vi "CRYAPI SPLITE LIB.vi"(4 "tSpliter_In":T3, 6 "tFrame":T2, 8 "tSpliter":T3, 9 "sData":string, 10 "nData":i32, 11 "sAction":string) -> (0 "nData_Out":i32, 2 "tFrame_Out":T2, 3 "tSpliter_Out":T3)   [LabVIEW 2013]
uses:
  <vilib>/Utility/miscctls.llb/LVRectTypeDef.ctl
  CRYMain Sub Window Global.vi
panel:
  out "sData_Out":string
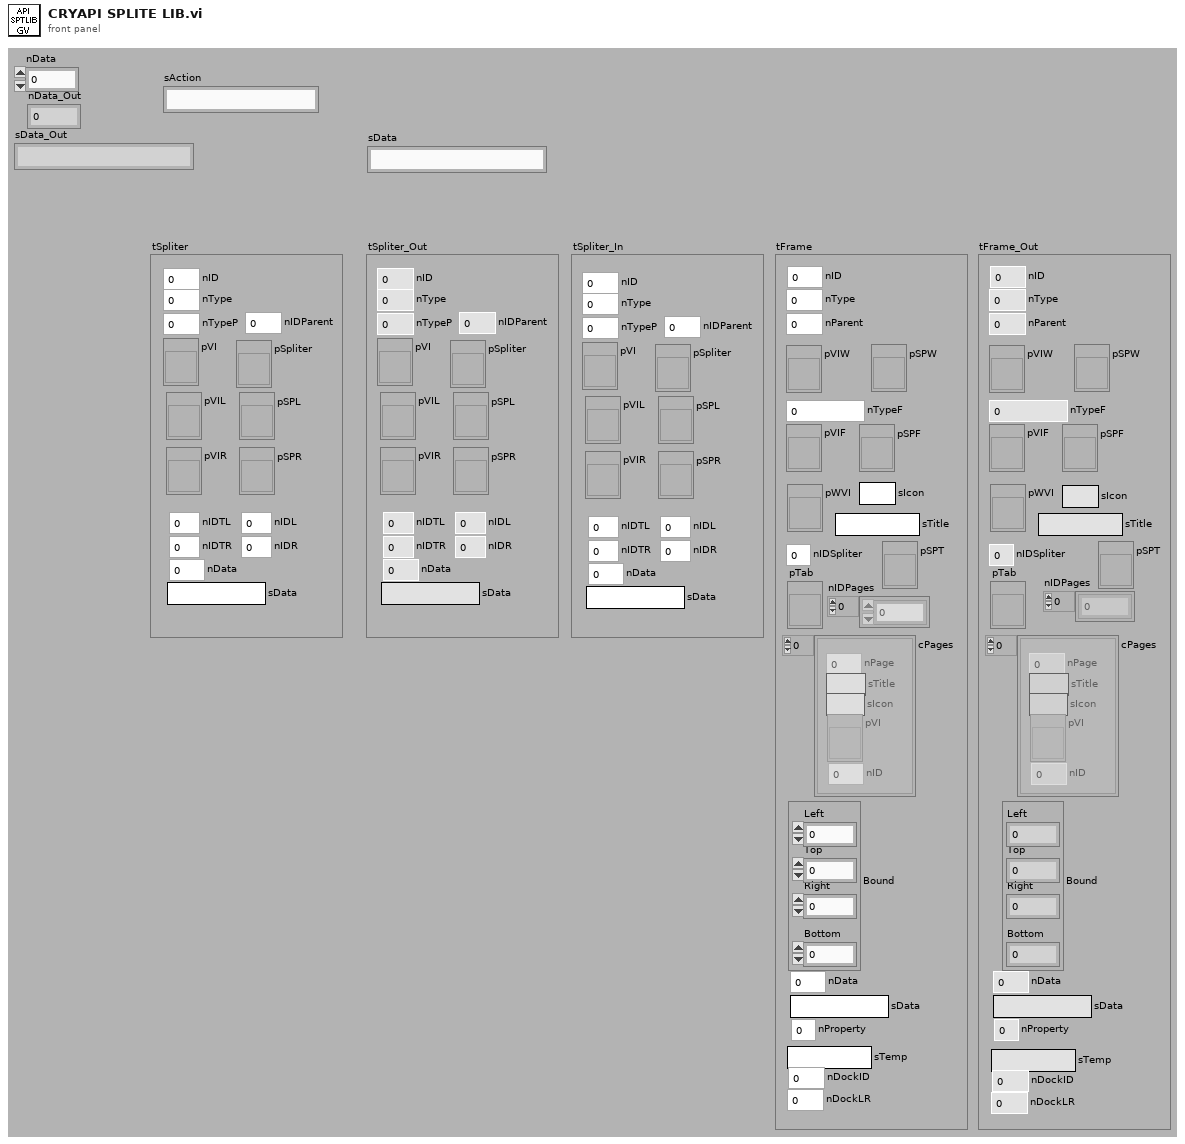
[diagram p1: front panel]
types:
  T1 = typedef "LVRectTypeDef.ctl" = cluster{"Left":i16, "Top":i16, "Right":i16, "Bottom":i16}
  T2 = cluster{"nType":i32, "nParent":i32, "pVIW":refnum<vi>, "pSPW":refnum<vi>, "nTypeF":i32, "pVIF":refnum<vi>, "pSPF":refnum<vi>, "nIDSpliter":i32, "nProperty":i32, "Bound":T1, "nID":i32, "nData":i32, "sData":string, "pWVI":refnum<vi>, "sTitle":string, "cPages":cluster{"nPage":i32, "sTitle":string, "sIcon":string, "pVI":refnum<vi>, "nID":i32}[], "pTab":refnum<vi>, "nIDPages":i32[], "pSPT":refnum<vi>, "sTemp":string, "nDockID":i32, "nDockLR":i32, "sIcon":string}
  T3 = cluster{"nType":i32, "nTypeP":i32, "pVI":refnum<vi>, "pSpliter":refnum<vi>, "pSPL":refnum<vi>, "pVIL":refnum<vi>, "pSPR":refnum<vi>, "pVIR":refnum<vi>, "nIDTL":i32, "nIDL":i32, "nIDTR":i32, "nIDR":i32, "nID":i32, "nIDParent":i32, "nData":i32, "sData":string}
  T4 = enum16{"Sticks Top/Left", "Sticks Bottom/Right", "Proportional"}
  T5 = enum32{"Invalid", "Standard", "Closed", "Hidden", "Minimized", "Maximized"}
  T6 = cluster{"pSP":refnum<vi>, "pVI":refnum<vi>, "nIDT":i32, "nID":i32, "nLR":i32}
  T7 = typedef "LVBoundsTypeDef.ctl" = cluster{"Width":u32, "Height":u32}
  T8 = cluster{"nID":i32[], "Spliter":cluster{"nType":i32, "nTypeP":i32, "pVI":refnum<vi>, "pSpliter":refnum<vi>, "pSPL":refnum<vi>, "pVIL":refnum<vi>, "pSPR":refnum<vi>, "pVIR":refnum<vi>, "nIDTL":i32, "nIDL":i32, "nIDTR":i32, "nIDR":i32, "nID":i32, "nIDParent":i32, "nData":i32, "sData":string}[]}
  T9 = cluster{"nType":i32, "nTypeP":i32, "pVI":refnum<vi>, "pSpliter":refnum<vi>, "pSPL":refnum<vi>, "pVIL":refnum<vi>, "pSPR":refnum<vi>, "pVIR":refnum<vi>, "nIDTL":i32, "nIDL":i32, "nIDTR":i32, "nIDR":i32, "nID":i32, "nIDParent":i32, "nData":i32, "sData":string}[]
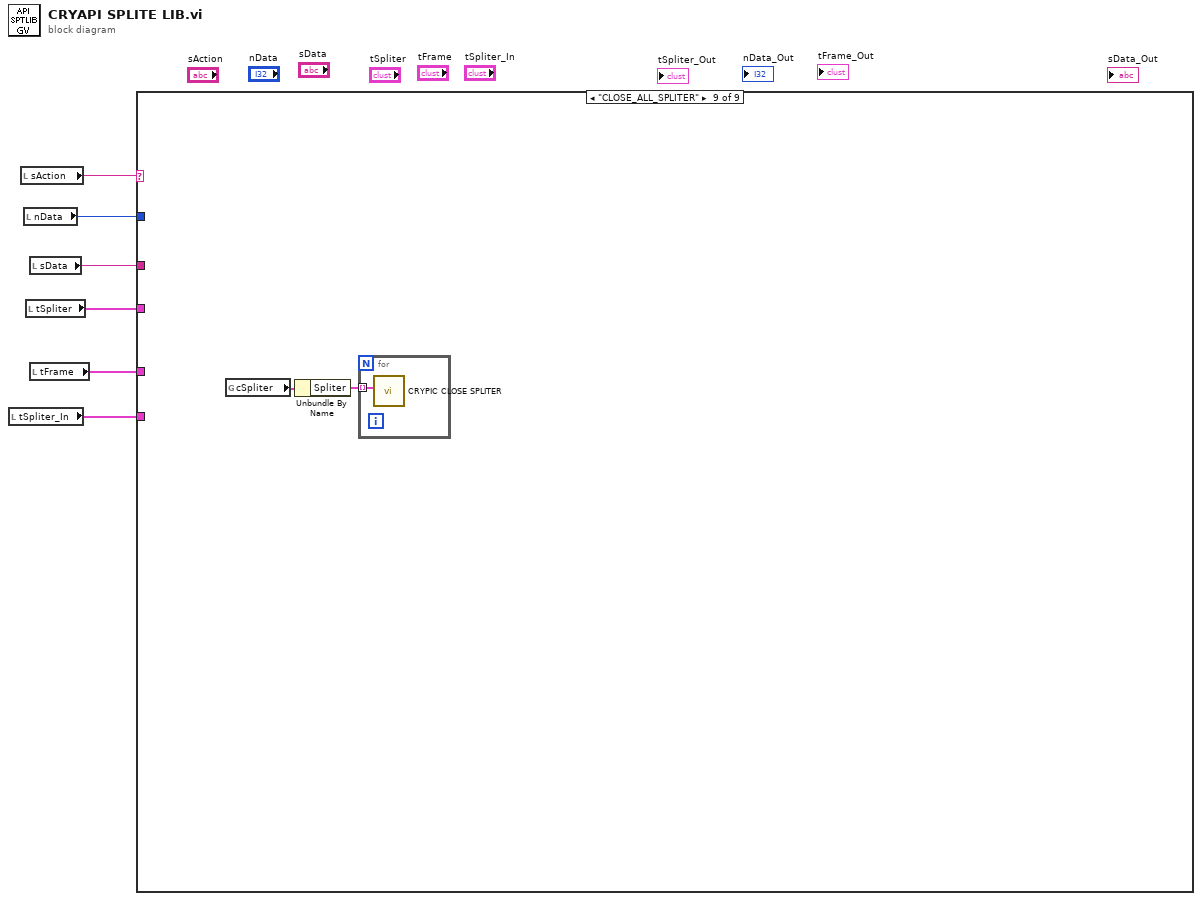
[diagram p0: block diagram]
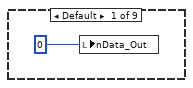
[diagram p2: hidden frame]
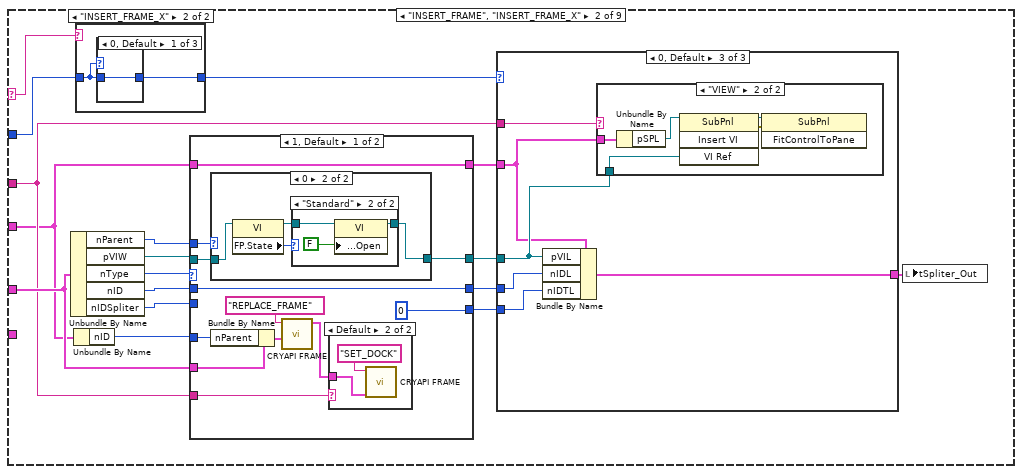
[diagram p3: hidden frame]
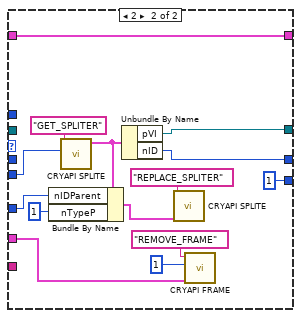
[diagram p7: hidden frame]
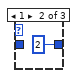
[diagram p9: hidden frame]
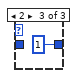
[diagram p10: hidden frame]
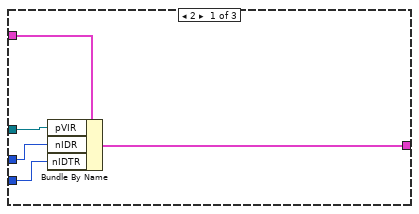
[diagram p11: hidden frame]
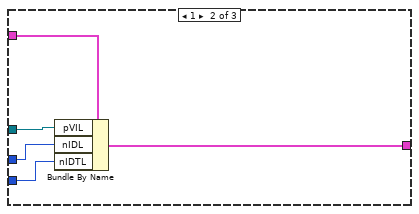
[diagram p12: hidden frame]
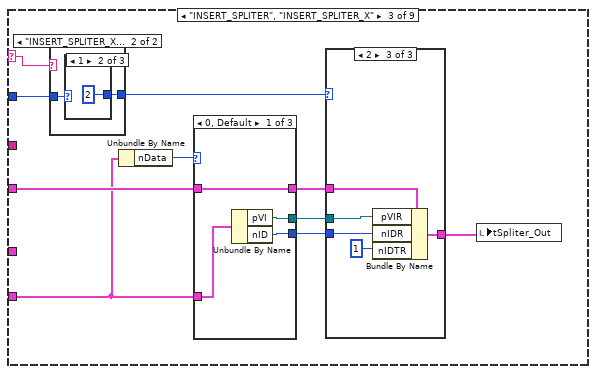
[diagram p14: hidden frame]
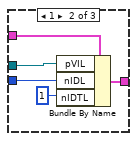
[diagram p16: hidden frame]
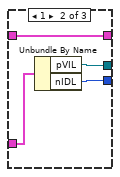
[diagram p17: hidden frame]
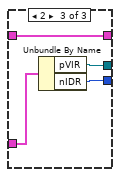
[diagram p18: hidden frame]
diagram:
  n1 = local read "tSpliter_In"() -> (w2:T3)
  n2 = local read "sAction"() -> (w6:string)
  n3 = local read "nData"() -> (w5:i32)
  n4 = local read "tSpliter"() -> (w1:T3)
  n5 = local read "sData"() -> (w3:string)
  n6 = local read "tFrame"() -> (w4:T2)
  n7 = case shown="\"CLOSE_ALL_SPLITER\"" w6 {
    selector: w6 -> [_ w16 w96 _ _ _ _ _ _]
    tunnel: w1 -> [_ w9 w97 w128 _ w391 _ _ _]
    tunnel: w5 -> [_ w15 w98 w130 w289 w392 w473 _ _]
    tunnel: w4 -> [_ w14 _ _ w291 w390 _ _ _]
    tunnel: w3 -> [_ w11 _ _ w290 _ _ _ _]
    tunnel: w2 -> [_ _ w90 w129 _ _ _ _ _]
    frame Default {
      n8 = local write "nData_Out"(0 ("nData_Out")) -> ()
    }
    frame "INSERT_FRAME", "INSERT_FRAME_X" {
      n9 = Unbundle By Name(w14) -> ("nParent"=w8:i32, "pVIW"=w12:refnum<vi>, "nType"=w22:i32, "nID"=w21:i32, "nIDSpliter"=w17:i32)
      n10 = Unbundle By Name(w9) -> ("nID"=w10:i32)
      n11 = case shown="\"INSERT_FRAME_X\"" w16 {
        tunnel: w15 -> [w62 w63]
        tunnel: [w62 w64] -> w23
        frame Default {
        }
        frame "INSERT_FRAME_X" {
          n12 = case shown="0, Default" w63 {
            tunnel: [w65 2 ("nData") 1 ("nData")] -> w64
            tunnel: w63 -> [w65 _ _]
            frame 0, Default {
            }
            frame 1 {
            }
            frame 2 {
            }
          }
        }
      }
      n13 = case shown="1, Default" w22 {
        tunnel: w21 -> [w32 _]
        tunnel: [w25 w58] -> w20
        tunnel: [w32 w57] -> w19
        tunnel: [0 ("nIDTR") 1 ("nIDTR")] -> w18
        tunnel: w17 -> [_ w59]
        tunnel: w14 -> [w33 w48]
        tunnel: w9 -> [w35 w54]
        tunnel: [w35 w54] -> w13
        tunnel: w10 -> [w31 w52]
        tunnel: w12 -> [w34 _]
        tunnel: w11 -> [w27 _]
        tunnel: w8 -> [w26 _]
        frame 1, Default {
          n14 = case shown="0" w26 {
            tunnel: w34 -> [w37 w39]
            tunnel: [w37 w38] -> w25
            frame Default {
            }
            frame 0 {
              n15 = property class="VI"(reference=w39) -> (reference out=w41:refnum<vi>, "FP.State"=w40:T5)  [unwired: 1 in, 1 out]
              n16 = case shown="\"Standard\"" w40 {
                tunnel: w41 -> [w42 w45]
                tunnel: [w42 w43] -> w38
                frame "Invalid", Default {
                }
                frame "Standard" {
                  n17 = property class="VI"(reference=w45, "Front Panel.Open"=FALSE ("Front Panel Window:Open")) -> (reference out=w43:refnum<vi>)  [unwired: 1 in, 1 out]
                }
              }
            }
          }
          n18 = Bundle By Name(cluster=w33, "nParent"=w31) -> (w29:T2)
          n19 = call "CRYAPI FRAME.vi"("tFrame"=w29, "sAction"="REPLACE_FRAME") -> ("tFrame_Out"=w28:T2)  [unwired: 4 in, 5 out]
          n20 = case shown="Default" w27 {
            tunnel: w28 -> [_ w46]
            frame "VIEW" {
            }
            frame Default {
              n21 = call "CRYAPI FRAME.vi"("tFrame"=w46, "sAction"="SET_DOCK") -> ()  [unwired: 4 in, 6 out]
            }
          }
        }
        frame 2 {
          n22 = call "CRYAPI SPLITE.vi"("nData"=w59, "sAction"="GET_SPLITER") -> ("tSpliter_Out"=w53:T3)  [unwired: 4 in, 5 out]
          n23 = Bundle By Name(cluster=w53, "nIDParent"=w52, "nTypeP"=1) -> (w49:T3)
          n24 = Unbundle By Name(w53) -> ("pVI"=w58:refnum<vi>, "nID"=w57:i32)
          n25 = call "CRYAPI SPLITE.vi"("tSpliter"=w49, "sAction"="REPLACE_SPLITER") -> ()  [unwired: 4 in, 6 out]
          n26 = call "CRYAPI FRAME.vi"("tFrame"=w48, "nData"=1, "sAction"="REMOVE_FRAME") -> ()  [unwired: 3 in, 6 out]
        }
      }
      n27 = case shown="0, Default" w23 {
        tunnel: [w72 w77 w81] -> w24
        tunnel: w20 -> [w71 w76 w79]
        tunnel: w19 -> [w70 w75 w83]
        tunnel: w18 -> [w68 w74 w82]
        tunnel: w13 -> [w69 w73 w78]
        tunnel: w11 -> [_ _ w80]
        frame 2 {
          n28 = Bundle By Name(cluster=w69, "pVIR"=w71, "nIDR"=w70, "nIDTR"=w68) -> (w72:T3)
        }
        frame 1 {
          n29 = Bundle By Name(cluster=w73, "pVIL"=w76, "nIDL"=w75, "nIDTL"=w74) -> (w77:T3)
        }
        frame 0, Default {
          n30 = Bundle By Name(cluster=w78, "pVIL"=w79, "nIDL"=w83, "nIDTL"=w82) -> (w81:T3)
          n31 = case shown="\"VIEW\"" w80 {
            tunnel: w79 -> [_ w84]
            tunnel: w78 -> [_ w88]
            frame Default {
            }
            frame "VIEW" {
              n32 = Unbundle By Name(w88) -> ("pSPL"=w87:refnum<vi>)
              n33 = invoke class="SubPnl" method="Insert VI"(reference=w87, "VI Ref"=w84) -> (reference out=w86:refnum<vi>, error out=w85:errorcluster)  [unwired: 2 in, 2 out]
              n34 = invoke class="SubPnl" method="FitControlToPane"(reference=w86, error in=w85) -> ()  [unwired: 1 in, 3 out]
            }
          }
        }
      }
      n35 = local write "tSpliter_Out"(w24) -> ()
    }
    frame "INSERT_SPLITER", "INSERT_SPLITER_X" {
      n36 = case shown="\"INSERT_SPLITER_X\"" w96 {
        tunnel: w98 -> [w122 w124]
        tunnel: [w122 w123] -> w95
        frame "INSERT_SPLITER", Default {
        }
        frame "INSERT_SPLITER_X" {
          n37 = case shown="1" w124 {
            selector: w124 -> [w125 _ _]
            tunnel: [w125 2 ("nData") 1 ("nData")] -> w123
            frame 0, Default {
            }
            frame 1 {
            }
            frame 2 {
            }
          }
        }
      }
      n38 = Unbundle By Name(w90) -> ("nData"=w89:i32)
      n39 = case shown="0, Default" w89 {
        tunnel: w97 -> [w112 w116 w120]
        tunnel: w90 -> [w113 w117 w121]
        tunnel: [w112 w116 w120] -> w94
        tunnel: [w111 w115 w119] -> w93
        tunnel: [w110 w114 w118] -> w92
        frame 0, Default {
          n40 = Unbundle By Name(w113) -> ("pVI"=w111:refnum<vi>, "nID"=w110:i32)
        }
        frame 1 {
          n41 = Unbundle By Name(w117) -> ("pVIL"=w115:refnum<vi>, "nIDL"=w114:i32)
        }
        frame 2 {
          n42 = Unbundle By Name(w121) -> ("pVIR"=w119:refnum<vi>, "nIDR"=w118:i32)
        }
      }
      n43 = case shown="2" w95 {
        tunnel: w94 -> [w99 w104 w109]
        tunnel: w93 -> [_ w102 w107]
        tunnel: w92 -> [_ w101 w106]
        tunnel: [w99 w100 w105] -> w91
        frame 0, Default {
        }
        frame 1 {
          n44 = Bundle By Name(cluster=w104, "pVIL"=w102, "nIDL"=w101, "nIDTL"=1) -> (w100:T3)
        }
        frame 2 {
          n45 = Bundle By Name(cluster=w109, "pVIR"=w107, "nIDR"=w106, "nIDTR"=1 ("nIDTL")) -> (w105:T3)
        }
      }
      n46 = local write "tSpliter_Out"(w91) -> ()
    }
    frame "MSIZE_SPLITER" {
      n47 = local write "tSpliter_Out"(w128) -> ()
      n48 = stacked-sequence {
        tunnel: w130 -> [w153 w250]
        tunnel: w129 -> [_ w261]
        tunnel: w128 -> [w152 w253]
        tunnel: w128 -> [w134 _]
        frame #0 {
          n49 = global read "CRYMain Sub Window Global.vi" "VritualVI"() -> (w138:refnum<vi>)
          n50 = Unbundle By Name(w134) -> ("nIDTL"=w133:i32, "nIDTR"=w132:i32)
          n51 = Unbundle By Name(w152) -> ("pVI"=w140:refnum<vi>)
          n52 = call "CRYAPI SPLITE.vi"("tSpliter"=w152, "nData"=w153, "sAction"="GET_LR_INDEX") -> ("tLR_Out"=w136:T6)  [unwired: 3 in, 5 out]
          n53 = Unbundle By Name(w136) -> ("pSP"=w135:refnum<vi>)
          n54 = Add(x=w133, y=w132) -> (x+y=w131:i32)
          n55 = property class="VI"(reference=w140) -> ("Front Panel.PanelBounds"=w139:T1)  [unwired: 1 in, 2 out]
          n56 = property class="VI"(reference=w138) -> ("Front Panel.PanelBounds"=w150:T1)  [unwired: 1 in, 2 out]
          n57 = property class="SubPnl"(reference=w135) -> ("Bounds"=w137:T7)  [unwired: 1 in, 2 out]
          n58 = Unbundle By Name(w152) -> ("nType"=w149:i32, "pSpliter"=w142:refnum<vi>)
          n59 = Unbundle By Name(w136) -> ("nIDT"=w147:i32)
          n60 = case shown="0, 1, Default" w149 {
            tunnel: w150 -> [w200 w225]
            tunnel: [w190 w215] -> w145
            tunnel: [w186 w211] -> w144
            tunnel: [w199 w224] -> w143
            tunnel: w153 -> [w198 w223]
            tunnel: [w198 w223] -> w148
            tunnel: w147 -> [w197 w222]
            tunnel: [w197 w222] -> w146
            tunnel: w142 -> [w196 w216]
            tunnel: [w196 w216] -> w141
            tunnel: w139 -> [w191 w217]
            tunnel: w137 -> [w189 w213]
            tunnel: w131 -> [w187 w212]
            frame 2 {
              n61 = Unbundle By Name(w200) -> ("Right"=w201:i16, "Left"=w202:i16, "Bottom"=w203:i16, "Top"=w204:i16)
              n62 = Unbundle By Name(w191) -> ("Right"=w195:i16, "Left"=w194:i16, "Bottom"=w193:i16, "Top"=w192:i16)
              n63 = Subtract(x=w201, y=w202) -> ()  [unwired: 1 out]
              n64 = Subtract(x=w203, y=w204) -> (x-y=w186:i16)
              n65 = case shown="Default" w187 {
                tunnel: w189 -> [_ w210]
                tunnel: [w206 w209] -> w188
                tunnel: w186 -> [w208 _]
                frame 0 {
                  n66 = Divide(x=w208, y=i16 2) -> (x/y=w205:dbl)
                  n67 = To Long Integer(number=w205) -> (32bit integer=w206:i32)
                }
                frame Default {
                  n68 = Unbundle By Name(w210) -> ("Height"=w209:u32)  [unwired: 1 out]
                }
              }
              n69 = Subtract(x=w195, y=w194) -> ()  [unwired: 1 out]
              n70 = Subtract(x=w193, y=w192) -> (x-y=w190:i16)
              n71 = Add(x=w186, y=w188) -> (x+y=w199:u32)
            }
            frame 0, 1, Default {
              n72 = Unbundle By Name(w225) -> ("Right"=w226:i16, "Left"=w227:i16, "Bottom"=w228:i16, "Top"=w229:i16)
              n73 = Unbundle By Name(w217) -> ("Right"=w221:i16, "Left"=w220:i16, "Bottom"=w219:i16, "Top"=w218:i16)
              n74 = Subtract(x=w226, y=w227) -> (x-y=w211:i16)
              n75 = case shown="Default" w212 {
                tunnel: w213 -> [_ w235]
                tunnel: [w230 w234] -> w214
                tunnel: w211 -> [w233 _]
                frame 0 {
                  n76 = Divide(x=w233, y=i16 2) -> (x/y=w231:dbl)
                  n77 = To Long Integer(number=w231) -> (32bit integer=w230:i32)
                }
                frame Default {
                  n78 = Unbundle By Name(w235) -> ("Width"=w234:u32)  [unwired: 1 out]
                }
              }
              n79 = Subtract(x=w228, y=w229) -> ()  [unwired: 1 out]
              n80 = Subtract(x=w221, y=w220) -> (x-y=w215:i16)
              n81 = Subtract(x=w219, y=w218) -> ()  [unwired: 1 out]
              n82 = Add(x=w211, y=w214) -> (x+y=w224:u32)
            }
          }
          n83 = case shown="0, Default" w146 {
            tunnel: w148 -> [_ w163]
            tunnel: w145 -> [_ w162]
            tunnel: w144 -> [_ w156]
            tunnel: w143 -> [_ w160]
            tunnel: w141 -> [_ w161]
            frame 1 {
              n84 = local write "nData_Out"(0 ("nData_Out")) -> ()
            }
            frame 0, Default {
              n85 = case shown="2" w163 {
                tunnel: w160 -> [w178 w185]
                tunnel: [w178 w182] -> w159
                tunnel: w162 -> [w177 w181]
                tunnel: [T4."Sticks Top/Left" ("Sizing") T4."Sticks Bottom/Right" ("Sizing")] -> w158
                tunnel: [w176 w183] -> w157
                tunnel: w156 -> [w175 w180]
                tunnel: [w175 w180] -> w155
                frame 0, 1, Default {
                  n86 = Less?(x=w178, y=w177) -> (x < y?=w176:bool)
                }
                frame 2 {
                  n87 = Subtract(x=w181, y=w185) -> (x-y=w182:u32)
                  n88 = Less?(x=w182, y=w181) -> (x < y?=w183:bool)
                }
              }
              n89 = case shown="True" w157 {
                tunnel: w161 -> [_ w170]
                tunnel: w159 -> [_ w167]
                tunnel: w158 -> [_ w169]
                tunnel: w155 -> [_ w165]
                frame False {
                  n90 = local write "nData_Out"(u32 0) -> ()
                }
                frame True {
                  n91 = property class="Splitter"(reference=w170, "Position"=w167) -> (reference out=w168:refnum<vi>, error out=w166:errorcluster)  [unwired: 1 in]
                  n92 = case shown="Error" w166 {
                    tunnel: w169 -> [w173 _]
                    tunnel: w168 -> [w172 _]
                    tunnel: w165 -> [w171 _]
                    frame No Error {
                      n93 = property class="Splitter"(reference=w172, "Sizing"=w173) -> ()  [unwired: 1 in, 2 out]
                      n94 = local write "nData_Out"(w171) -> ()
                    }
                    frame Error {
                      n95 = local write "nData_Out"(0 ("nData_Out")) -> ()
                    }
                  }
                }
              }
            }
          }
        }
        frame #1 {
          w237 = i16 0 ("Left")
          n96 = local read "nData_Out"() -> (w256:i32)
          n97 = Unbundle By Name(w261) -> ("nType"=w248:i32, "pSpliter"=w255:refnum<vi>, "pVI"=w244:refnum<vi>)
          n98 = call "CRYAPI SPLITE.vi"("tSpliter"=w253, "nData"=w250, "sAction"="GET_LR_INDEX") -> ("tLR_Out"=w252:T6)  [unwired: 3 in, 5 out]
          n99 = Unbundle By Name(w252) -> ("pSP"=w251:refnum<vi>)
          n100 = property class="SubPnl"(reference=w251) -> ("Bounds"=w240:T7)  [unwired: 1 in, 2 out]
          n101 = Unbundle By Name(w240) -> ("Width"=w239:u32, "Height"=w238:u32)
          n102 = case shown="0, 1, Default" w248 {
            tunnel: w240 -> [w265 w267]
            tunnel: [w264 w266] -> w247
            frame 2 {
              n103 = Unbundle By Name(w265) -> ("Height"=w264:u32)  [unwired: 1 out]
            }
            frame 0, 1, Default {
              n104 = Unbundle By Name(w267) -> ("Width"=w266:u32)  [unwired: 1 out]
            }
          }
          n105 = Bundle By Name(cluster=T1 {"Left"=0, "Top"=0, "Right"=0, "Bottom"=0} ("Front Panel Window:Panel Bounds"), "Left"=w237, "Top"=w237, "Right"=w239, "Bottom"=w238) -> (w241:T1)
          n106 = property class="VI"(reference=w244, "Front Panel.PanelBounds"=w241) -> (reference out=w243:refnum<vi>)  [unwired: 1 in, 1 out]
          n107 = case shown="0" w256 {
            selector: w256 -> [_ w277]
            tunnel: w255 -> [w268 w274]
            tunnel: w250 -> [w271 w278]
            tunnel: [w271 w278] -> w249
            tunnel: [w270 w275] -> w245
            tunnel: w247 -> [w269 w276]
            tunnel: [w268 w274] -> w246
            tunnel: w243 -> [_ _]
            frame 0 {
              n108 = Divide(x=w269, y=i16 2) -> (x/y=w272:dbl)
              n109 = To Long Integer(number=w272) -> (32bit integer=w270:i32)
            }
            frame Default {
              n110 = case shown="2" w278 {
                tunnel: w277 -> [w279 w281]
                tunnel: w276 -> [_ w282]
                tunnel: [w279 w280] -> w275
                frame 0, 1, Default {
                }
                frame 2 {
                  n111 = Subtract(x=w282, y=w281) -> (x-y=w280:u32)
                }
              }
            }
          }
          n112 = case shown="2" w249 {
            tunnel: [w283 w286] -> w259
            tunnel: w246 -> [w285 w288]
            tunnel: [w285 w288] -> w258
            tunnel: [T4."Sticks Top/Left" ("Sizing") T4."Sticks Top/Left" ("Sizing")] -> w257
            tunnel: w245 -> [w283 w286]
            frame 0, 1, Default {
            }
            frame 2 {
            }
          }
          n113 = property class="Splitter"(reference=w258, "Position"=w259) -> (reference out=w260:refnum<vi>, error out=w236:errorcluster)  [unwired: 1 in]
          n114 = case shown="No Error" w236 {
            tunnel: w260 -> [w263 _]
            tunnel: w257 -> [w262 _]
            frame No Error {
              n115 = property class="Splitter"(reference=w263, "Sizing"=w262) -> ()  [unwired: 1 in, 2 out]
            }
            frame Error {
            }
          }
        }
      }
    }
    frame "GET_SPLITER_WIN" {
      n116 = Unbundle By Name(w291) -> ("nIDSpliter"=w295:i32)
      n117 = case shown="\"VSPLITER\"" w290 {
        tunnel: [0 2 1 0] -> w292
        frame Default {
        }
        frame "HSPLITER" {
        }
        frame "VSPLITER" {
        }
        frame "NSPLITER" {
        }
      }
      n118 = call "CRYAPI SPLITE.vi"("nData"=w295, "sAction"="GET_SPLITER") -> ("tSpliter_Out"=w293:T3)  [unwired: 4 in, 5 out]
      n119 = Unbundle By Name(w293) -> ("nType"=w294:i32)
      n120 = Equal?(x=w292, y=w294) -> (x = y?=w296:bool)
      n121 = case shown="True" w296 {
        tunnel: w289 -> [_ w308]
        tunnel: w295 -> [_ w307]
        tunnel: w293 -> [w299 _]
        tunnel: w292 -> [_ w300]
        frame False {
          n122 = local write "nData_Out"(-1 ("nData_Out")) -> ()
          n123 = local write "tSpliter_Out"(w299) -> ()
        }
        frame True {
          n124 = while {
            shift-right: [w366] -> w306
            shift-left: w307 -> [w368]
            tunnel: w308 -> [w362]
            tunnel: [w363] -> w310
            tunnel: [w362] -> w305
            tunnel: w300 -> [w361]
            stop <- w367 stop-if-true
            n125 = call "CRYAPI SPLITE.vi"("nData"=w368, "sAction"="GET_SPLITER") -> ("tSpliter_Out"=w364:T3)  [unwired: 4 in, 5 out]
            n126 = Unbundle By Name(w364) -> ("nType"=w365:i32)
            n127 = case shown="1, 2" w365 {
              selector: w365 -> [_ w377]
              tunnel: w362 -> [_ w384]
              tunnel: w364 -> [_ w383]
              tunnel: [TRUE w375] -> w367
              tunnel: [-1 ("nID") w379] -> w366
              tunnel: w364 -> [w370 w378]
              tunnel: [w370 w378] -> w363
              tunnel: w361 -> [_ w376]
              frame 0, Default {
              }
              frame 1, 2 {
                n128 = Equal?(x=w377, y=w376) -> (x = y?=w373:bool)
                n129 = call "CRYAPI SPLITE.vi"("tSpliter"=w383, "nData"=w384, "sAction"="GET_LR_INDEX") -> ("tLR_Out"=w382:T6)  [unwired: 3 in, 5 out]
                n130 = Unbundle By Name(w382) -> ("nIDT"=w381:i32, "nID"=w379:i32)
                n131 = Equal?(x=0, y=w381) -> (x = y?=w374:bool)
                n132 = And(x=w374, y=w373) -> (x .and. y?=w375:bool)
              }
            }
          }
          n133 = Unbundle By Name(w310) -> ("nType"=w312:i32)
          n134 = Equal?(x=0, y=w312) -> (x = y?=w309:bool)
          n135 = case shown="True" w309 {
            selector: w309 -> [_ w355]
            tunnel: [w320 w355] -> w302
            tunnel: w310 -> [w324 _]
            frame False {
              n136 = Unbundle By Name(w324) -> ("nIDTL"=w328:i32, "nIDTR"=w327:i32, "nType"=w323:i32, "pSPL"=w322:refnum<vi>, "pSPR"=w321:refnum<vi>)
              n137 = case shown="1, Default" w323 {
                tunnel: w322 -> [w341 w354]
                tunnel: w321 -> [w340 w353]
                tunnel: [w329 w342] -> w319
                frame 1, Default {
                  n138 = property class="SubPnl"(reference=w340) -> ("Width"=w338:u32)  [unwired: 1 in, 2 out]
                  n139 = property class="SubPnl"(reference=w341) -> ("Width"=w339:u32)  [unwired: 1 in, 2 out]
                  n140 = global read "CRYMain Sub Window Global.vi" "VritualVI"() -> (w332:refnum<vi>)
                  n141 = property class="VI"(reference=w332) -> ("Front Panel.PanelBounds"=w333:T1)  [unwired: 1 in, 2 out]
                  n142 = Add(x=w339, y=w338) -> (x+y=w330:u32)
                  n143 = Unbundle By Name(w333) -> ("Right"=w334:i16, "Left"=w335:i16, "Bottom"=w336:i16, "Top"=w337:i16)
                  n144 = Subtract(x=w334, y=w335) -> (x-y=w331:i16)
                  n145 = Subtract(x=w336, y=w337) -> ()  [unwired: 1 out]
                  n146 = Less?(x=w330, y=w331) -> (x < y?=w329:bool)
                }
                frame 2 {
                  n147 = property class="SubPnl"(reference=w353) -> ("Height"=w351:u32)  [unwired: 1 in, 2 out]
                  n148 = property class="SubPnl"(reference=w354) -> ("Height"=w352:u32)  [unwired: 1 in, 2 out]
                  n149 = global read "CRYMain Sub Window Global.vi" "VritualVI"() -> (w346:refnum<vi>)
                  n150 = property class="VI"(reference=w346) -> ("Front Panel.PanelBounds"=w345:T1)  [unwired: 1 in, 2 out]
                  n151 = Add(x=w352, y=w351) -> (x+y=w343:u32)
                  n152 = Unbundle By Name(w345) -> ("Right"=w347:i16, "Left"=w348:i16, "Bottom"=w349:i16, "Top"=w350:i16)
                  n153 = Subtract(x=w347, y=w348) -> ()  [unwired: 1 out]
                  n154 = Subtract(x=w349, y=w350) -> (x-y=w344:i16)
                  n155 = Less?(x=w343, y=w344) -> (x < y?=w342:bool)
                }
              }
              n156 = Add(x=w328, y=w327) -> (x+y=w326:i32)
              n157 = Equal?(x=w326, y=0) -> (x = y?=w318:bool)
              n158 = And(x=w318, y=w319) -> (x .and. y?=w320:bool)
            }
            frame True {
            }
          }
          n159 = case shown="Default" w306 {
            selector: w306 -> [_ w316]
            tunnel: w305 -> [w315 _]
            tunnel: [w315 w316] -> w304
            tunnel: [FALSE TRUE] -> w301
            frame Default {
            }
            frame -1 {
            }
          }
          n160 = Or(x=w301, y=w302) -> (x .or. y?=w303:bool)
          n161 = case shown="True" w303 {
            tunnel: w310 -> [w356 _]
            tunnel: [w356 w358] -> w311
            tunnel: w307 -> [_ w359]
            frame False {
            }
            frame True {
              n162 = local write "nData_Out"(-1 ("nData_Out")) -> ()
              n163 = call "CRYAPI SPLITE.vi"("nData"=w359, "sAction"="GET_SPLITER") -> ("tSpliter_Out"=w358:T3)  [unwired: 4 in, 5 out]
            }
          }
          n164 = local write "tSpliter_Out"(w311) -> ()
          n165 = local write "nData_Out"(w304) -> ()
        }
      }
    }
    frame "EXCHANGE_FRAME_LR" {
      n166 = case shown="2" w392 {
        tunnel: w391 -> [w413 w450]
        tunnel: w390 -> [w412 w449]
        frame 0, 1, Default {
          n167 = stacked-sequence {
            tunnel: w413 -> [w428]
            tunnel: [w428] -> w411
            tunnel: w412 -> [w427]
            tunnel: [w427] -> w410
            tunnel: [w426] -> w401
            frame #0 {
              n168 = Unbundle By Name(w428) -> ("nIDL"=w426:i32, "pSPL"=w429:refnum<vi>)
              n169 = invoke class="SubPnl" method="Remove VI"(reference=w429) -> ()  [unwired: 2 in, 3 out]
            }
          }
          n170 = stacked-sequence {
            tunnel: w411 -> [w422]
            tunnel: w410 -> [w423]
            tunnel: [w423] -> w409
            tunnel: [w422] -> _
            tunnel: [w421] -> w400
            frame #0 {
              n171 = Unbundle By Name(w423) -> ("pVIW"=w420:refnum<vi>, "nID"=w425:i32)
              n172 = Bundle By Name(cluster=w422, "nIDTL"=0 ("nIDT"), "pVIL"=w420, "nIDL"=w425) -> (w421:T3)
            }
          }
          n173 = call "CRYAPI FRAME.vi"("nData"=w401, "sAction"="GET_FRAME") -> ("tFrame_Out"=w407:T2)  [unwired: 4 in, 5 out]
          n174 = Bundle By Name(cluster=w407, "nParent"=0) -> (w404:T2)
          n175 = call "CRYAPI FRAME.vi"("tFrame"=w404, "sAction"="REPLACE_FRAME") -> ("tFrame_Out"=w402:T2)  [unwired: 4 in, 5 out]
          n176 = call "CRYAPI FRAME.vi"("tFrame"=w402, "sAction"="SET_DOCK") -> ("tFrame_Out"=w393:T2)  [unwired: 4 in, 5 out]
          n177 = stacked-sequence {
            tunnel: w400 -> [w417]
            tunnel: w409 -> [w418]
            tunnel: [w418] -> _
            tunnel: [w417] -> w396
            tunnel: [w419] -> w395
            frame #0 {
              n178 = Unbundle By Name(w417) -> ("nID"=w416:i32, "pSPL"=w415:refnum<vi>, "pVIL"=w414:refnum<vi>)
              n179 = invoke class="SubPnl" method="Insert VI"(reference=w415, "VI Ref"=w414) -> ()  [unwired: 2 in, 4 out]
              n180 = Bundle By Name(cluster=w418, "nParent"=w416) -> (w419:T2)
            }
          }
          n181 = Unbundle By Name(w393) -> ("nID"=w394:i32)
          n182 = local write "nData_Out"(w394) -> ()
          n183 = local write "tFrame_Out"(w395) -> ()
          n184 = local write "tSpliter_Out"(w396) -> ()
          n185 = call "CRYAPI FRAME.vi"("tFrame"=w395, "sAction"="SET_DOCK") -> ()  [unwired: 4 in, 6 out]
          n186 = call "CRYAPI SPLITE.vi"("tSpliter"=w396, "sAction"="REPLACE_SPLITER") -> ()  [unwired: 4 in, 6 out]
          n187 = call "CRYAPI FRAME.vi"("tFrame"=w395, "sAction"="REPLACE_FRAME") -> ()  [unwired: 4 in, 6 out]
        }
        frame 2 {
          n188 = stacked-sequence {
            tunnel: w450 -> [w465]
            tunnel: [w465] -> w448
            tunnel: w449 -> [w464]
            tunnel: [w464] -> w447
            tunnel: [w463] -> w437
            frame #0 {
              n189 = Unbundle By Name(w465) -> ("nIDR"=w463:i32, "pSPR"=w466:refnum<vi>)
              n190 = invoke class="SubPnl" method="Remove VI"(reference=w466) -> ()  [unwired: 2 in, 3 out]
            }
          }
          n191 = stacked-sequence {
            tunnel: w448 -> [w459]
            tunnel: w447 -> [w460]
            tunnel: [w460] -> w446
            tunnel: [w458] -> w434
            frame #0 {
              n192 = Unbundle By Name(w460) -> ("pVIW"=w457:refnum<vi>, "nID"=w462:i32)
              n193 = Bundle By Name(cluster=w459, "nIDTR"=0 ("nIDT"), "pVIR"=w457, "nIDR"=w462) -> (w458:T3)
            }
          }
          n194 = call "CRYAPI FRAME.vi"("nData"=w437, "sAction"="GET_FRAME") -> ("tFrame_Out"=w444:T2)  [unwired: 4 in, 5 out]
          n195 = Bundle By Name(cluster=w444, "nParent"=0) -> (w441:T2)
          n196 = call "CRYAPI FRAME.vi"("tFrame"=w441, "sAction"="REPLACE_FRAME") -> ("tFrame_Out"=w439:T2)  [unwired: 4 in, 5 out]
          n197 = call "CRYAPI FRAME.vi"("tFrame"=w439, "sAction"="SET_DOCK") -> ("tFrame_Out"=w431:T2)  [unwired: 4 in, 5 out]
          n198 = stacked-sequence {
            tunnel: w434 -> [w454]
            tunnel: w446 -> [w455]
            tunnel: [w455] -> _
            tunnel: [w454] -> w435
            tunnel: [w456] -> w432
            frame #0 {
              n199 = Unbundle By Name(w454) -> ("nID"=w453:i32, "pSPR"=w452:refnum<vi>, "pVIR"=w451:refnum<vi>)
              n200 = invoke class="SubPnl" method="Insert VI"(reference=w452, "VI Ref"=w451) -> ()  [unwired: 2 in, 4 out]
              n201 = Bundle By Name(cluster=w455, "nParent"=w453) -> (w456:T2)
            }
          }
          n202 = Unbundle By Name(w431) -> ("nID"=w430:i32)
          n203 = local write "nData_Out"(w430) -> ()
          n204 = local write "tFrame_Out"(w432) -> ()
          n205 = local write "tSpliter_Out"(w435) -> ()
          n206 = call "CRYAPI FRAME.vi"("tFrame"=w432, "sAction"="SET_DOCK") -> ()  [unwired: 4 in, 6 out]
          n207 = call "CRYAPI FRAME.vi"("tFrame"=w432, "sAction"="REPLACE_FRAME") -> ()  [unwired: 4 in, 6 out]
          n208 = call "CRYAPI SPLITE.vi"("tSpliter"=w435, "sAction"="REPLACE_SPLITER") -> ()  [unwired: 4 in, 6 out]
        }
      }
    }
    frame "CHECK_ROOT" {
      n209 = while {
        shift-right: [w481] -> w471
        shift-left: w473 -> [w485]
        tunnel: [w480] -> w468
        stop <- w482 stop-if-true
        n210 = call "CRYAPI SPLITE.vi"("nData"=w485, "sAction"="GET_SPLITER") -> ("tSpliter_Out"=w479:T3)  [unwired: 4 in, 5 out]
        n211 = Unbundle By Name(w479) -> ("nTypeP"=w484:i32, "nIDParent"=w481:i32, "nType"=w480:i32)
        n212 = Equal?(x=0, y=w484) -> (x = y?=w482:bool)
      }
      n213 = call "CRYAPI FRAME.vi"("nData"=w471, "sAction"="GET_FRAME") -> ("tFrame_Out"=w467:T2)  [unwired: 4 in, 5 out]
      n214 = Unbundle By Name(w467) -> ("nType"=w470:i32)
      n215 = local write "tFrame_Out"(w467) -> ()
      n216 = case shown="0, Default" w470 {
        tunnel: [w475 1 ("x")] -> w469
        tunnel: w468 -> [w474 _]
        frame 0, Default {
          n217 = case shown="Default" w474 {
            tunnel: [1 ("x") 0 ("x")] -> w475
            frame 0 {
            }
            frame Default {
            }
          }
        }
        frame 1, 2 {
        }
      }
      n218 = local write "nData_Out"(w469) -> ()
    }
    frame "DETACH_ALL_SPLITER" {
      n219 = global read "CRYMain Sub Window Global.vi" "cSpliter"() -> (w488:T8)
      n220 = Unbundle By Name(w488) -> ("Spliter"=w487:T9)
      n221 = for {
        tunnel: w487 -> [w489] mode=indexing
        n222 = Unbundle By Name(w489) -> ("nType"=w490:i32)
        n223 = case shown="1, 2" w490 {
          tunnel: w489 -> [w492 w494]
          frame 0, Default {
            n224 = Unbundle By Name(w492) -> ("pSPL"=w491:refnum<vi>)
            n225 = invoke class="SubPnl" method="Remove VI"(reference=w491) -> ()  [unwired: 2 in, 3 out]
          }
          frame 1, 2 {
            n226 = Unbundle By Name(w494) -> ("pSPL"=w495:refnum<vi>, "pSPR"=w493:refnum<vi>)
            n227 = invoke class="SubPnl" method="Remove VI"(reference=w495) -> ()  [unwired: 2 in, 3 out]
            n228 = invoke class="SubPnl" method="Remove VI"(reference=w493) -> ()  [unwired: 2 in, 3 out]
          }
        }
      }
    }
    frame "CLOSE_ALL_SPLITER" {
      n229 = global read "CRYMain Sub Window Global.vi" "cSpliter"() -> (w497:T8)
      n230 = Unbundle By Name(w497) -> ("Spliter"=w496:T9)
      n231 = for {
        tunnel: w496 -> [w498] mode=indexing
        n232 = call "CRYPIC CLOSE SPLITER.vi"("tSpliter"=w498) -> ()  [unwired: 10 in, 1 out]
      }
    }
  }
